vi "NumIntegrate_Rkf45_NEW.vi"(4 "MaxTruncError":dbl, 5 "Func_X_U_Extra":T1, 6 "dT_Remaining":dbl, 7 "PassedData":variant, 8 "InitialH":dbl, 10 "U":T2, 11 "X":T2) -> (0 "Error":bool, 1 "IterationCount":i32, 2 "H":dbl, 3 "NewX":T2)   [LabVIEW 2019]
doc: "Implements one loop of RKF45. This takes an initial state, dt guess, and max truncation error, and returns a new x and the dt over which that x was updated. This should be called until there is no dt remaining.\n\nThis is an INTERNAL FUNCTION AND SHOULD NOT BE CALLED DIRECTLY.\n\n\n * @return the integration of dx/dt = f(x, u) for dt.\n */\n\n\nInputs:\n - Func_X_U_Extra -- A strictly typed LabVIEW reference to a function to integrate as a function of matrix X, U, and the extra passed data\n - PassedData -- This is a variant that can be used to pass additional data to the function if needed. The data must be packed into the variant in the specific way expected by the function.\n - X -- The initial value of x.\n - U -- The value u held constant over the integration period.\n - InitialH -- The initial dt guess. This is refined to clamp truncation error to the specified max.\n - dT_Remaining -- How much time is left to integrate over. Used to clamp h.\n - Max TruncError -- The max truncation error acceptable. Usually a small number like 1e-6.\n\nOutputs:\n - New X -- the integration of dx/dt = f(x, u) for dt\n - H -- \n - Iteration count -- How many times this routine looped to achieve the desired error tolerance\n - Error -- If TRUE, an error occured."
uses:
  Trajectory_Library.lvlib
  <vilib>/Analysis/Matrix/NI_Matrix.lvlib
  <vilib>/Analysis/Matrix/Numeric/Multiply/Multiply - RM,R.vi
  <vilib>/Analysis/Matrix/Numeric/Add/Add - RM,RM.vi
  <vilib>/Analysis/NI_AALPro.lvlib
  <vilib>/Analysis/_algsub.llb/Real Matrix Norm.vi
  <vilib>/Analysis/_algsub.llb/Matrix Norm Type.ctl
  <vilib>/Analysis/Matrix/Datatypes/RealMatrix.ctl
  CALLBACK_FUNC_TYPE.ctl
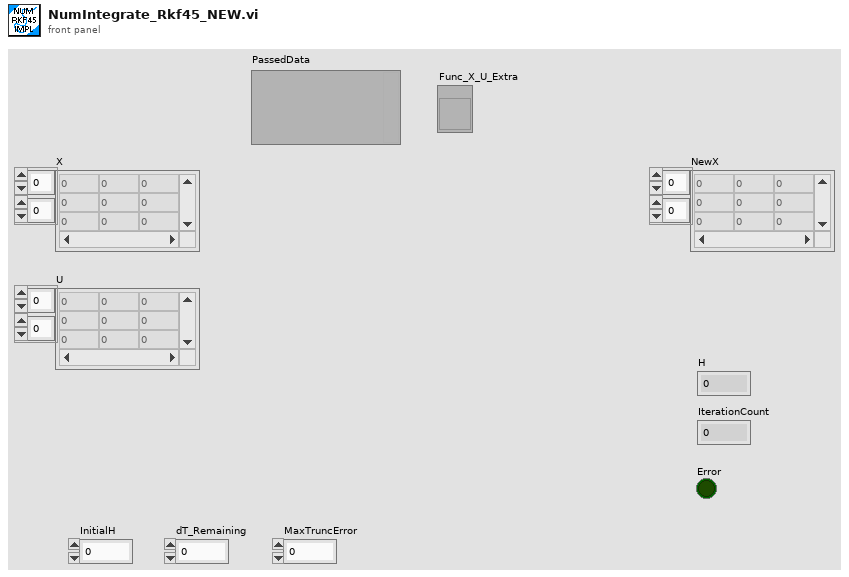
[diagram p1: front panel]
types:
  T1 = typedef "Trajectory_Library.lvlib/CALLBACK_FUNC_TYPE.ctl" = refnum<vi>
  T2 = typedef "NI_Matrix.lvlib/RealMatrix.ctl" = dbl[][]
  T3 = typedef "NI_AALPro.lvlib/Matrix Norm Type.ctl" = i32
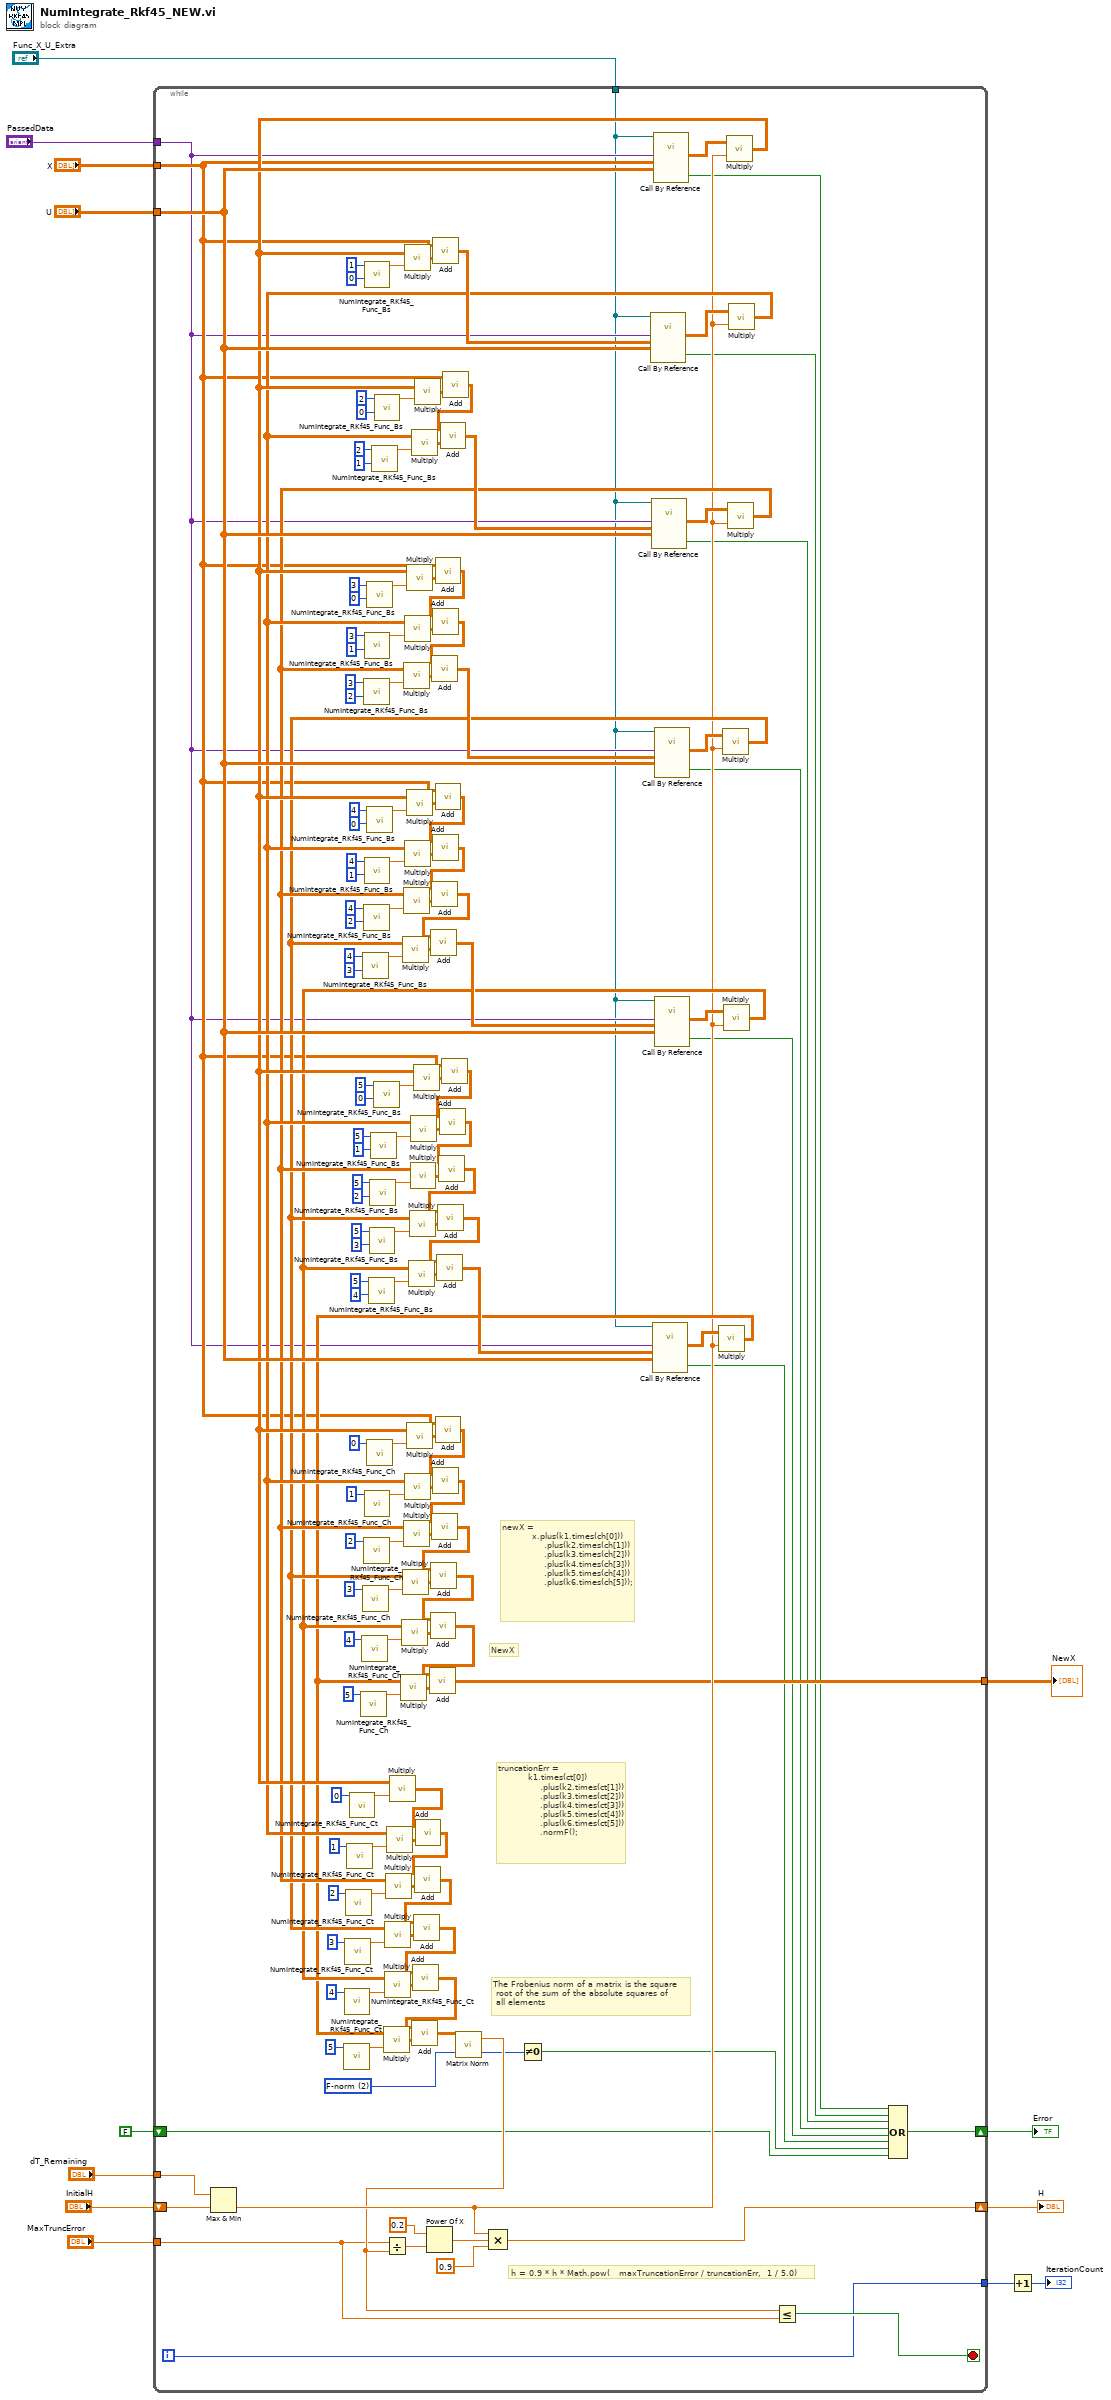
[diagram p0: block diagram]
diagram:
  n1 = while {
    tunnel: "PassedData" -> [w25]
    shift-right: [w35] -> w8
    shift-left: "InitialH" -> [w34]
    tunnel: "X" -> [w26]
    tunnel: "U" -> [w173]
    tunnel: "MaxTruncError" -> [w30]
    tunnel: "dT_Remaining" -> [w33]
    tunnel: [w28] -> w5
    tunnel: [w27] -> w7
    tunnel: "Func_X_U_Extra" -> [w24]
    shift-right: [w14] -> w1
    shift-left: FALSE -> [w23]
    i -> [w27]
    stop <- w29 stop-if-true
    w40 = T3 2 items=["2-norm", "1-norm", "F-norm", "Inf-norm"] ("norm type")
    # "h = 0.9 * h * Math.pow(   maxTruncationError / truncationErr,  1 / 5.0)"
    # "The Frobenius norm of a matrix is the square\n root of the sum of the absolute squares of\n all elements"
    # "truncationErr =\n          k1.times(ct[0])\n              .plus(k2.times(ct[1]))\n              .plus(k3.times(ct[2]))\n              .plus(k4.times(ct[3]))\n              .plus(k5.times(ct[4]))\n              .plus(k6.times(ct[5]))\n              .normF();"
    # "NewX"
    # "newX =\n          x.plus(k1.times(ch[0]))\n              .plus(k2.times(ch[1]))\n              .plus(k3.times(ch[2]))\n              .plus(k4.times(ch[3]))\n              .plus(k5.times(ch[4]))\n              .plus(k6.times(ch[5]));"
    n2 = Max & Min(x=w33, y=w34) -> (min(x,y)=w32:dbl)  [unwired: 1 out]
    n3 = call "NumIntegrate_RKf45_Func_Ct.vi"("Index"=5 ("Row")) -> ("Ct"=w52:dbl)  [unwired: 10 in]
    n4 = call "NumIntegrate_RKf45_Func_Ct.vi"("Index"=4 ("Row")) -> ("Ct"=w56:dbl)  [unwired: 10 in]
    n5 = call "NumIntegrate_RKf45_Func_Ct.vi"("Index"=3 ("Row")) -> ("Ct"=w60:dbl)  [unwired: 10 in]
    n6 = call "NumIntegrate_RKf45_Func_Ct.vi"("Index"=2 ("Row")) -> ("Ct"=w64:dbl)  [unwired: 10 in]
    n7 = call "NumIntegrate_RKf45_Func_Ct.vi"("Index"=1 ("Row")) -> ("Ct"=w67:dbl)  [unwired: 10 in]
    n8 = call "NumIntegrate_RKf45_Func_Ct.vi"("Index"=0 ("Row")) -> ("Ct"=w69:dbl)  [unwired: 10 in]
    n9 = call "NumIntegrate_RKf45_Func_Ch.vi"("Index"=5 ("Row")) -> ("Ch"=w73:dbl)  [unwired: 10 in]
    n10 = call "NumIntegrate_RKf45_Func_Ch.vi"("Index"=4 ("Row")) -> ("Ch"=w77:dbl)  [unwired: 10 in]
    n11 = call "NumIntegrate_RKf45_Func_Bs.vi"("Col"=3, "Row"=4) -> ("Bs"=w123:dbl)  [unwired: 9 in]
    n12 = call "NumIntegrate_RKf45_Func_Ch.vi"("Index"=3 ("Row")) -> ("Ch"=w81:dbl)  [unwired: 10 in]
    n13 = call "NumIntegrate_RKf45_Func_Bs.vi"("Col"=2, "Row"=3) -> ("Bs"=w143:dbl)  [unwired: 9 in]
    n14 = call "NumIntegrate_RKf45_Func_Bs.vi"("Col"=2, "Row"=4) -> ("Bs"=w128:dbl)  [unwired: 9 in]
    n15 = call "NumIntegrate_RKf45_Func_Ch.vi"("Index"=2 ("Row")) -> ("Ch"=w85:dbl)  [unwired: 10 in]
    n16 = call "NumIntegrate_RKf45_Func_Bs.vi"("Col"=0, "Row"=1) -> ("Bs"=w167:dbl)  [unwired: 9 in]
    n17 = call "NumIntegrate_RKf45_Func_Bs.vi"("Col"=1, "Row"=3) -> ("Bs"=w148:dbl)  [unwired: 9 in]
    n18 = call "NumIntegrate_RKf45_Func_Bs.vi"("Col"=1, "Row"=4) -> ("Bs"=w133:dbl)  [unwired: 9 in]
    n19 = call "NumIntegrate_RKf45_Func_Ch.vi"("Index"=1 ("Row")) -> ("Ch"=w89:dbl)  [unwired: 10 in]
    n20 = call "NumIntegrate_RKf45_Func_Bs.vi"("Col"=0, "Row"=3) -> ("Bs"=w152:dbl)  [unwired: 9 in]
    n21 = call "NumIntegrate_RKf45_Func_Bs.vi"("Col"=0, "Row"=4) -> ("Bs"=w137:dbl)  [unwired: 9 in]
    n22 = call "NumIntegrate_RKf45_Func_Ch.vi"("Index"=0 ("Row")) -> ("Ch"=w92:dbl)  [unwired: 10 in]
    n23 = call "NumIntegrate_RKf45_Func_Bs.vi"("Col"=4, "Row"=5) -> ("Bs"=w98:dbl)  [unwired: 9 in]
    n24 = call "NumIntegrate_RKf45_Func_Bs.vi"("Col"=3, "Row"=5) -> ("Bs"=w103:dbl)  [unwired: 9 in]
    n25 = call "NumIntegrate_RKf45_Func_Bs.vi"("Col"=2, "Row"=5) -> ("Bs"=w108:dbl)  [unwired: 9 in]
    n26 = call "NumIntegrate_RKf45_Func_Bs.vi"("Col"=1, "Row"=5) -> ("Bs"=w113:dbl)  [unwired: 9 in]
    n27 = call "NumIntegrate_RKf45_Func_Bs.vi"("Col"=1, "Row"=2) -> ("Bs"=w158:dbl)  [unwired: 9 in]
    n28 = call "NumIntegrate_RKf45_Func_Bs.vi"("Col"=0, "Row"=5) -> ("Bs"=w117:dbl)  [unwired: 9 in]
    n29 = call "NumIntegrate_RKf45_Func_Bs.vi"("Col"=0, "Row"=2) -> ("Bs"=w162:dbl)  [unwired: 9 in]
    n30 = call-by-ref "?"(reference=w24, "U"=w173, "X"=w26, "Variant"=w25) -> ("Error"=w15:bool, "NewX"=w174:T2)  [unwired: 8 in, 2 out]
    n31 = call-poly <vilib>:"Multiply.vi"("Real Scalar c"=w32, "Real Matrix A"=w174) -> ("A * c"=w48:T2)
    n32 = call-poly <vilib>:"Multiply.vi"("Real Scalar c"=w69, "Real Matrix A"=w48) -> ("A * c"=w47:T2)
    n33 = call-poly <vilib>:"Multiply.vi"("Real Scalar c"=w167, "Real Matrix A"=w48) -> ("A * c"=w166:T2)
    n34 = call-poly <vilib>:"Multiply.vi"("Real Scalar c"=w152, "Real Matrix A"=w48) -> ("A * c"=w151:T2)
    n35 = call-poly <vilib>:"Multiply.vi"("Real Scalar c"=w137, "Real Matrix A"=w48) -> ("A * c"=w136:T2)
    n36 = call-poly <vilib>:"Multiply.vi"("Real Scalar c"=w92, "Real Matrix A"=w48) -> ("A * c"=w91:T2)
    n37 = call-poly <vilib>:"Multiply.vi"("Real Scalar c"=w117, "Real Matrix A"=w48) -> ("A * c"=w116:T2)
    n38 = call-poly <vilib>:"Multiply.vi"("Real Scalar c"=w162, "Real Matrix A"=w48) -> ("A * c"=w161:T2)
    n39 = call-poly <vilib>:"Add.vi"("Real Matrix B"=w166, "Real Matrix A"=w26) -> ("A + B"=w165:T2)
    n40 = call-poly <vilib>:"Add.vi"("Real Matrix B"=w151, "Real Matrix A"=w26) -> ("A + B"=w144:T2)
    n41 = call-poly <vilib>:"Add.vi"("Real Matrix B"=w136, "Real Matrix A"=w26) -> ("A + B"=w129:T2)
    n42 = call-poly <vilib>:"Add.vi"("Real Matrix B"=w91, "Real Matrix A"=w26) -> ("A + B"=w86:T2)
    n43 = call-poly <vilib>:"Add.vi"("Real Matrix B"=w116, "Real Matrix A"=w26) -> ("A + B"=w109:T2)
    n44 = call-poly <vilib>:"Add.vi"("Real Matrix B"=w161, "Real Matrix A"=w26) -> ("A + B"=w154:T2)
    n45 = call-by-ref "?"(reference=w24, "U"=w173, "X"=w165, "Variant"=w25) -> ("Error"=w16:bool, "NewX"=w168:T2)  [unwired: 8 in, 2 out]
    n46 = call-poly <vilib>:"Multiply.vi"("Real Scalar c"=w32, "Real Matrix A"=w168) -> ("A * c"=w46:T2)
    n47 = call-poly <vilib>:"Multiply.vi"("Real Scalar c"=w67, "Real Matrix A"=w46) -> ("A * c"=w66:T2)
    n48 = call-poly <vilib>:"Multiply.vi"("Real Scalar c"=w148, "Real Matrix A"=w46) -> ("A * c"=w147:T2)
    n49 = call-poly <vilib>:"Multiply.vi"("Real Scalar c"=w133, "Real Matrix A"=w46) -> ("A * c"=w132:T2)
    n50 = call-poly <vilib>:"Multiply.vi"("Real Scalar c"=w89, "Real Matrix A"=w46) -> ("A * c"=w88:T2)
    n51 = call-poly <vilib>:"Multiply.vi"("Real Scalar c"=w113, "Real Matrix A"=w46) -> ("A * c"=w112:T2)
    n52 = call-poly <vilib>:"Multiply.vi"("Real Scalar c"=w158, "Real Matrix A"=w46) -> ("A * c"=w157:T2)
    n53 = call-poly <vilib>:"Add.vi"("Real Matrix B"=w66, "Real Matrix A"=w47) -> ("A + B"=w61:T2)
    n54 = call-poly <vilib>:"Add.vi"("Real Matrix B"=w147, "Real Matrix A"=w144) -> ("A + B"=w139:T2)
    n55 = call-poly <vilib>:"Add.vi"("Real Matrix B"=w132, "Real Matrix A"=w129) -> ("A + B"=w124:T2)
    n56 = call-poly <vilib>:"Add.vi"("Real Matrix B"=w88, "Real Matrix A"=w86) -> ("A + B"=w82:T2)
    n57 = call-poly <vilib>:"Add.vi"("Real Matrix B"=w112, "Real Matrix A"=w109) -> ("A + B"=w104:T2)
    n58 = call-poly <vilib>:"Add.vi"("Real Matrix B"=w157, "Real Matrix A"=w154) -> ("A + B"=w153:T2)
    n59 = call-by-ref "?"(reference=w24, "U"=w173, "X"=w153, "Variant"=w25) -> ("Error"=w17:bool, "NewX"=w169:T2)  [unwired: 8 in, 2 out]
    n60 = call-poly <vilib>:"Multiply.vi"("Real Scalar c"=w32, "Real Matrix A"=w169) -> ("A * c"=w45:T2)
    n61 = call-poly <vilib>:"Multiply.vi"("Real Scalar c"=w64, "Real Matrix A"=w45) -> ("A * c"=w63:T2)
    n62 = call-poly <vilib>:"Multiply.vi"("Real Scalar c"=w143, "Real Matrix A"=w45) -> ("A * c"=w142:T2)
    n63 = call-poly <vilib>:"Multiply.vi"("Real Scalar c"=w128, "Real Matrix A"=w45) -> ("A * c"=w127:T2)
    n64 = call-poly <vilib>:"Multiply.vi"("Real Scalar c"=w85, "Real Matrix A"=w45) -> ("A * c"=w84:T2)
    n65 = call-poly <vilib>:"Multiply.vi"("Real Scalar c"=w108, "Real Matrix A"=w45) -> ("A * c"=w107:T2)
    n66 = call-poly <vilib>:"Add.vi"("Real Matrix B"=w63, "Real Matrix A"=w61) -> ("A + B"=w57:T2)
    n67 = call-poly <vilib>:"Add.vi"("Real Matrix B"=w142, "Real Matrix A"=w139) -> ("A + B"=w138:T2)
    n68 = call-poly <vilib>:"Add.vi"("Real Matrix B"=w127, "Real Matrix A"=w124) -> ("A + B"=w119:T2)
    n69 = call-poly <vilib>:"Add.vi"("Real Matrix B"=w84, "Real Matrix A"=w82) -> ("A + B"=w78:T2)
    n70 = call-poly <vilib>:"Add.vi"("Real Matrix B"=w107, "Real Matrix A"=w104) -> ("A + B"=w99:T2)
    n71 = call-by-ref "?"(reference=w24, "U"=w173, "X"=w138, "Variant"=w25) -> ("Error"=w18:bool, "NewX"=w170:T2)  [unwired: 8 in, 2 out]
    n72 = call-poly <vilib>:"Multiply.vi"("Real Scalar c"=w32, "Real Matrix A"=w170) -> ("A * c"=w44:T2)
    n73 = call-poly <vilib>:"Multiply.vi"("Real Scalar c"=w60, "Real Matrix A"=w44) -> ("A * c"=w59:T2)
    n74 = call-poly <vilib>:"Multiply.vi"("Real Scalar c"=w123, "Real Matrix A"=w44) -> ("A * c"=w122:T2)
    n75 = call-poly <vilib>:"Multiply.vi"("Real Scalar c"=w81, "Real Matrix A"=w44) -> ("A * c"=w80:T2)
    n76 = call-poly <vilib>:"Multiply.vi"("Real Scalar c"=w103, "Real Matrix A"=w44) -> ("A * c"=w102:T2)
    n77 = call-poly <vilib>:"Add.vi"("Real Matrix B"=w59, "Real Matrix A"=w57) -> ("A + B"=w53:T2)
    n78 = call-poly <vilib>:"Add.vi"("Real Matrix B"=w122, "Real Matrix A"=w119) -> ("A + B"=w118:T2)
    n79 = call-poly <vilib>:"Add.vi"("Real Matrix B"=w80, "Real Matrix A"=w78) -> ("A + B"=w74:T2)
    n80 = call-poly <vilib>:"Add.vi"("Real Matrix B"=w102, "Real Matrix A"=w99) -> ("A + B"=w94:T2)
    n81 = call-by-ref "?"(reference=w24, "U"=w173, "X"=w118, "Variant"=w25) -> ("Error"=w19:bool, "NewX"=w171:T2)  [unwired: 8 in, 2 out]
    n82 = call-poly <vilib>:"Multiply.vi"("Real Scalar c"=w32, "Real Matrix A"=w171) -> ("A * c"=w43:T2)
    n83 = call-poly <vilib>:"Multiply.vi"("Real Scalar c"=w56, "Real Matrix A"=w43) -> ("A * c"=w55:T2)
    n84 = call-poly <vilib>:"Multiply.vi"("Real Scalar c"=w77, "Real Matrix A"=w43) -> ("A * c"=w76:T2)
    n85 = call-poly <vilib>:"Multiply.vi"("Real Scalar c"=w98, "Real Matrix A"=w43) -> ("A * c"=w97:T2)
    n86 = call-poly <vilib>:"Add.vi"("Real Matrix B"=w55, "Real Matrix A"=w53) -> ("A + B"=w49:T2)
    n87 = call-poly <vilib>:"Add.vi"("Real Matrix B"=w76, "Real Matrix A"=w74) -> ("A + B"=w70:T2)
    n88 = call-poly <vilib>:"Add.vi"("Real Matrix B"=w97, "Real Matrix A"=w94) -> ("A + B"=w93:T2)
    n89 = call-by-ref "?"(reference=w24, "U"=w173, "X"=w93, "Variant"=w25) -> ("Error"=w20:bool, "NewX"=w172:T2)  [unwired: 8 in, 2 out]
    n90 = call-poly <vilib>:"Multiply.vi"("Real Scalar c"=w32, "Real Matrix A"=w172) -> ("A * c"=w42:T2)
    n91 = call-poly <vilib>:"Multiply.vi"("Real Scalar c"=w52, "Real Matrix A"=w42) -> ("A * c"=w51:T2)
    n92 = call-poly <vilib>:"Multiply.vi"("Real Scalar c"=w73, "Real Matrix A"=w42) -> ("A * c"=w72:T2)
    n93 = call-poly <vilib>:"Add.vi"("Real Matrix B"=w51, "Real Matrix A"=w49) -> ("A + B"=w41:T2)
    n94 = call-poly <vilib>:"Add.vi"("Real Matrix B"=w72, "Real Matrix A"=w70) -> ("A + B"=w28:T2)
    n95 = call-poly <vilib>:"Matrix Norm.vi"("norm type"=w40, "Input Matrix"=w41) -> ("error"=w22:i32, "norm"=w31:dbl)
    n96 = Divide(x=w30, y=w31) -> (x/y=w38:dbl)
    n97 = Power Of X(1:w38, 2:0.2 ("x")) -> (0:w37:dbl)
    n98 = Compound Arithmetic op=MULTIPLY(w32, w37, 0.9 ("value")) -> (w35:dbl)
    n99 = Not Equal To 0?(x=w22) -> (x != 0?=w21:bool)
    n100 = Less Or Equal?(x=w31, y=w30) -> (x <= y?=w29:bool)
    n101 = Compound Arithmetic op=OR(w15, w16, w17, w18, w19, w20, w21, w23) -> (w14:bool)
  }
  "NewX" <- w5
  "H" <- w8
  "Error" <- w1
  n102 = Increment(x=w7) -> (x+1=→"IterationCount":i32)
